vi "_Fade(I32).vi"(6 "Fade (Exponential)":T1, 8 "error in":errorcluster, 9 "Target Transparency (0)":u8, 10 "Fade time (ms)":i32, 11 "VI Reference (calling VI)":refnum<vi>) -> (0 "error out":errorcluster, 3 "dup VI Reference":refnum<vi>)   [LabVIEW 2012]
doc: "Produces a fade in or out, from the actual value to the target transparency. Use this generic VI when you start from an unknown transparency value."
uses:
  _fadetype.ctl
  SetTransparency(U8).vi
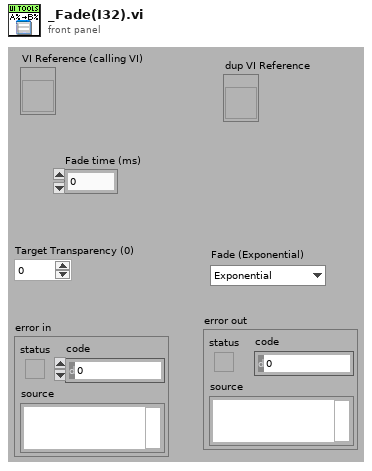
[diagram p1: front panel]
types:
  T1 = typedef "_fadetype.ctl" = enum16{"Exponential", "Linear"}
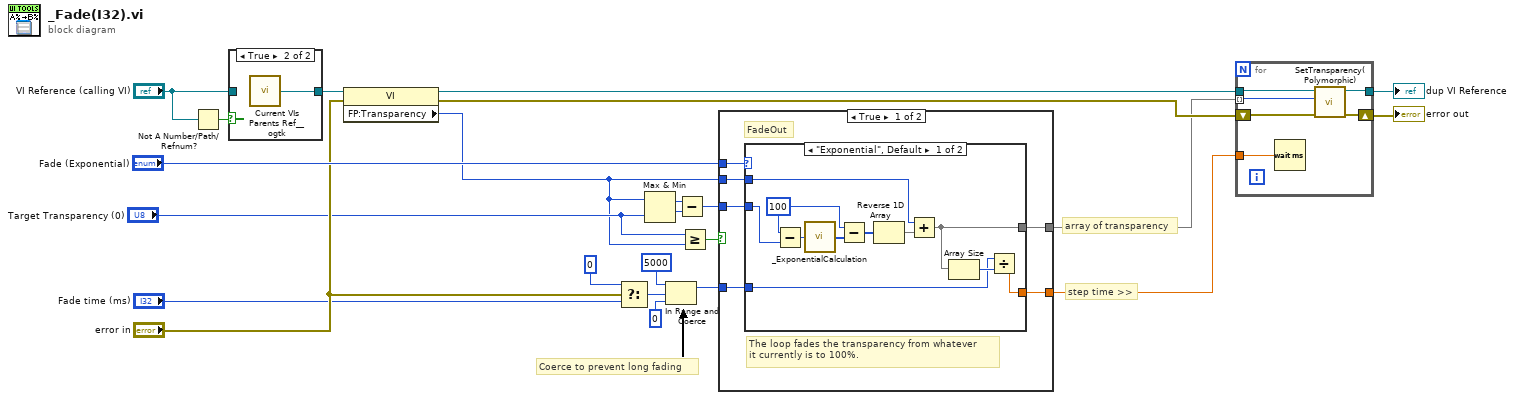
[diagram p0: block diagram]
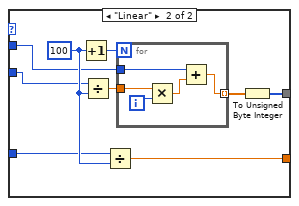
[diagram p2: hidden frame]
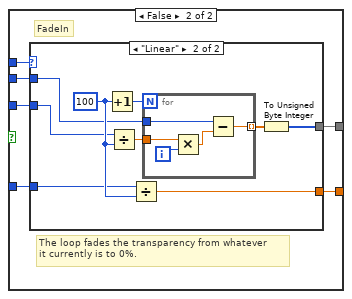
[diagram p3: hidden frame]
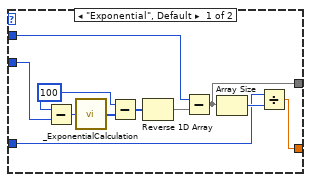
[diagram p4: hidden frame]
diagram:
  # "array of transparency"
  # "step time >>"
  # "Coerce to prevent long fading"
  n1 = Not A Number/Path/Refnum?(number/path/refnum="VI Reference (calling VI)") -> (NaN/Path/Refnum?=w23:bool)
  n2 = case shown="True" w23 {
    tunnel: "VI Reference (calling VI)" -> [w24 _]
    tunnel: [w24 w25] -> w15
    frame False {
    }
    frame True {
      n3 = call <userlib>:"Current VIs Parents Ref__ogtk.vi"() -> ("Calling VI's Reference"=w25:refnum<vi>)  [unwired: 2 out]
    }
  }
  n4 = property class="VI"(reference=w15, error in="error in") -> (reference out=w9:refnum<vi>, error out=w8:errorcluster, "FP:Transparency"=w1:u8)
  n5 = Select(t=0 ("output 1"), s="error in", f="Fade time (ms)") -> (s? t:f=w20:i32)
  n6 = Max & Min(x=w1, y="Target Transparency (0)") -> (max(x,y)=w2:u8, min(x,y)=w4:u8)
  n7 = In Range and Coerce(upper limit=5000 ("output 1"), x=w20, lower limit=0 ("output 1")) -> (coerced(x)=w17:i32)  [unwired: 1 out]
  n8 = Subtract(x=w2, y=w4) -> (x-y=w3:u8)
  n9 = Greater Or Equal?(x="Target Transparency (0)", y=w1) -> (x >= y?=w16:bool)
  n10 = case shown="True" w16 {
    tunnel: w17 -> [w29 w60]
    tunnel: w1 -> [w31 w62]
    tunnel: "Fade (Exponential)" -> [w30 w61]
    tunnel: [w28 w59] -> w7
    tunnel: [w27 w58] -> w6
    tunnel: w3 -> [w26 w57]
    frame True {
      # "FadeOut"
      # "The loop fades the transparency from whatever\nit currently is to 100%."
      n11 = case shown="\"Exponential\", Default" w30 {
        tunnel: w31 -> [w33 w43]
        tunnel: w29 -> [w41 w47]
        tunnel: [w32 w46] -> w27
        tunnel: [w34 w45] -> w28
        tunnel: w26 -> [w37 w44]
        frame "Exponential", Default {
          w38 = u8 100 ("x")
          n12 = Subtract(x=w38, y=w37) -> (x-y=w40:u8)
          n13 = call "_ExponentialCalculation.vi"("Initial FP:Transparency"=w40) -> ("Transparency Array"=w39:u8[])
          n14 = Subtract(x=w38, y=w39) -> (x-y=w36:u8[])
          n15 = Reverse 1D Array(array=w36) -> (reversed array=w35:u8[])
          n16 = Add(x=w33, y=w35) -> (x+y=w34:u8[])
          n17 = Array Size(array=w34) -> (size(s)=w42:i32)
          n18 = Divide(x=w41, y=w42) -> (x/y=w32:dbl)
        }
        frame "Linear" {
          w48 = 100
          n19 = Increment(x=w48) -> (x+1=w50:i32)
          n20 = Divide(x=w44, y=w48) -> (x/y=w51:dbl)
          n21 = Divide(x=w47, y=w48) -> (x/y=w46:dbl)
          n22 = for {
            N: w50 -> [_]
            tunnel: w51 -> [w55]
            tunnel: [w52] -> w49 mode=indexing
            tunnel: w43 -> [w54]
            i -> [w56]
            n23 = Multiply(x=w55, y=w56) -> (x*y=w53:dbl)
            n24 = Add(x=w54, y=w53) -> (x+y=w52:dbl)
          }
          n25 = To Unsigned Byte Integer(number=w49) -> (unsigned 8bit integer=w45:u8[])
        }
      }
    }
    frame False {
      # "FadeIn"
      # "The loop fades the transparency from whatever\nit currently is to 0%."
      n26 = case shown="\"Linear\"" w61 {
        tunnel: w62 -> [w66 w74]
        tunnel: w60 -> [w72 w76]
        tunnel: [w71 w78] -> w58
        tunnel: [w65 w77] -> w59
        tunnel: w57 -> [w63 w75]
        frame "Exponential", Default {
          w70 = u8 100 ("x")
          n27 = Subtract(x=w70, y=w63) -> (x-y=w69:u8)
          n28 = call "_ExponentialCalculation.vi"("Initial FP:Transparency"=w69) -> ("Transparency Array"=w68:u8[])
          n29 = Subtract(x=w70, y=w68) -> (x-y=w67:u8[])
          n30 = Reverse 1D Array(array=w67) -> (reversed array=w64:u8[])
          n31 = Subtract(x=w66, y=w64) -> (x-y=w65:u8[])
          n32 = Array Size(array=w65) -> (size(s)=w73:i32)
          n33 = Divide(x=w72, y=w73) -> (x/y=w71:dbl)
        }
        frame "Linear" {
          w79 = 100
          n34 = Increment(x=w79) -> (x+1=w81:i32)
          n35 = Divide(x=w75, y=w79) -> (x/y=w82:dbl)
          n36 = Divide(x=w76, y=w79) -> (x/y=w78:dbl)
          n37 = for {
            N: w81 -> [_]
            tunnel: w82 -> [w86]
            tunnel: [w83] -> w80 mode=indexing
            tunnel: w74 -> [w85]
            i -> [w87]
            n38 = Multiply(x=w86, y=w87) -> (x*y=w84:dbl)
            n39 = Subtract(x=w85, y=w84) -> (x-y=w83:dbl)
          }
          n40 = To Unsigned Byte Integer(number=w80) -> (unsigned 8bit integer=w77:u8[])
        }
      }
    }
  }
  n41 = for {
    tunnel: w9 -> [w92]
    tunnel: w6 -> [w93]
    tunnel: [w88] -> w11
    shift-right: [w89] -> w10
    shift-left: w8 -> [w90]
    tunnel: w7 -> [w91] mode=indexing
    n42 = Wait (ms)(milliseconds to wait=w93) -> ()  [unwired: 1 out]
    n43 = call-poly "SetTransparency(Polymorphic).vi"("error in"=w90, "Transparency (%)"=w91, "VI Reference (calling VI)"=w92) -> ("error out"=w89:errorcluster, "dup VI Reference"=w88:refnum<vi>)  [unwired: 1 in, 6 out]
  }
  "dup VI Reference" <- w11
  "error out" <- w10
